vi "Create Channel.vi"(6 "index":i32, 8 "error in":errorcluster, 10 "settings":T1, 11 "PWM Mode in":refnum<class "PWM Mode.lvclass">) -> (0 "error out":errorcluster, 2 "PWM channel out":refnum<class "PWM Output Channel.lvclass">, 3 "PWM Mode out":refnum<class "PWM Mode.lvclass">)   [LabVIEW 2017, in "Scan Engine Scripting.lvlib" / "PWM Mode.lvclass"]
uses:
  PWM Mode.lvclass
  Controls/pwm channel settings.ctl
  Channel Classes/PWM Output Channel/Frequency.ctl
  Channel Classes/PWM Output Channel/PWM Output Channel.lvclass
  PWM Mode.lvclass/PWM Mode.ctl
  Scan Engine Scripting.lvlib
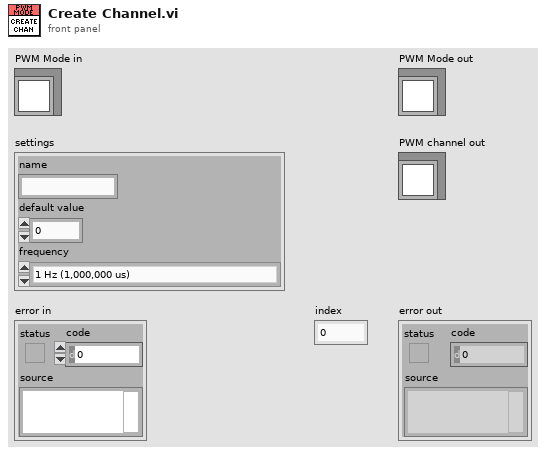
[diagram p1: front panel]
types:
  T1 = typedef "Scan Engine Scripting.lvlib/pwm channel settings.ctl" = cluster{"name":string, "default value":dbl, "frequency":T2}
  T2 = typedef "Scan Engine Scripting.lvlib/PWM Output Channel.lvclass/Frequency.ctl" = enum16{"1 Hz (1,000,000 us)", "50 Hz (20,000 us)", "250 Hz (4,000 us)", "500 Hz (2,000 us)", "1 kHz (1,000 us)", "5 kHz (200 us)", "10 kHz (100 us)", "20 kHz (50 us)"}
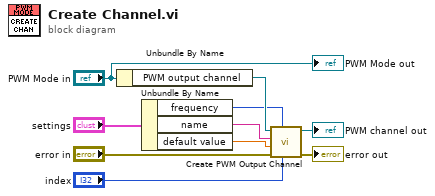
[diagram p0: block diagram]
diagram:
  n1 = Unbundle By Name("PWM Mode in") -> ("PWM output channel"=w2:refnum<class "PWM Output Channel.lvclass">)
  n2 = Unbundle By Name("settings") -> ("frequency"=w1:T2, "name"=w4:string, "default value"=w3:dbl)
  n3 = call "Create PWM Output Channel.vi"("index"="index", "frequency"=w1, "error in"="error in", "default value"=w3, "name"=w4, "PWM channel in"=w2) -> ("error out"=→"error out":errorcluster, "PWM channel out"=→"PWM channel out":refnum<class "PWM Output Channel.lvclass">)  [unwired: 4 in]
  "PWM Mode out" <- "PWM Mode in"
